vi "Call Subpanel VI.vi"(8 "error in (no error)":errorcluster, 10 "VI Refnum":refnum<vi>, 11 "DispSnsr Configuration in":refnum<class "DispSnsr Configuration.lvclass">) -> (0 "error out":errorcluster, 3 "DispSnsr Configuration out":refnum<class "DispSnsr Configuration.lvclass">)   [LabVIEW 2016, in "Hardware.lvlib" / "Displacement Sensor.lvlib" / "DispSnsr Configuration.lvclass"]
uses:
  <userlib>/Common Components/Hardware/Displacement Sensor/DispSnsr Config/DispSnsr Configuration.lvclass
  <userlib>/Configuration Dialog Actor/Configuration.lvclass
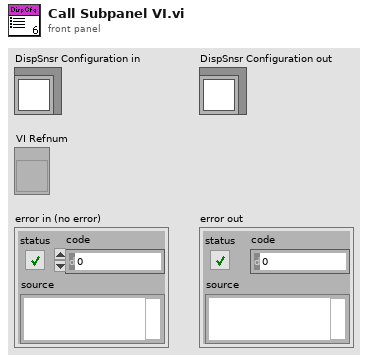
[diagram p1: front panel]
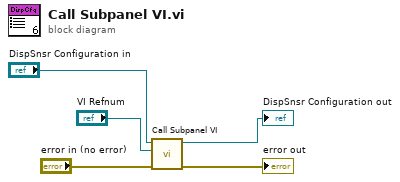
[diagram p0: block diagram]
diagram:
  n1 = call-parent "Call Subpanel VI.vi"("error in (no error)"="error in (no error)", "VI Refnum"="VI Refnum", "Configuration in"="DispSnsr Configuration in") -> ("error out"=→"error out":errorcluster, "Configuration out"=→"DispSnsr Configuration out":refnum<class "DispSnsr Configuration.lvclass">)  [unwired: 7 in]
